vi "Read Bytes by Value.vi"(8 "Error In":errorcluster, 10 "Count":u64, 11 "Reader In":refnum<class "Reader.lvclass">) -> (0 "Error Out":errorcluster, 2 "Bytes":u8[](array[numeric]), 3 "Reader Out":refnum<class "Reader.lvclass">)   [LabVIEW 2018, in "Toolkit.lvlib" / "Reader.lvclass"]
uses:
  Reader.lvclass
  Reader.lvclass/Reader.ctl
  Public/Status/Read Status.vi
  Public/Status/Read Status Message.vi
  Public/Status/Read Is Error.vi
  Utility/Status Code.vi
  <vilib>/Utility/error.llb/Error Cluster From Error Code.vi
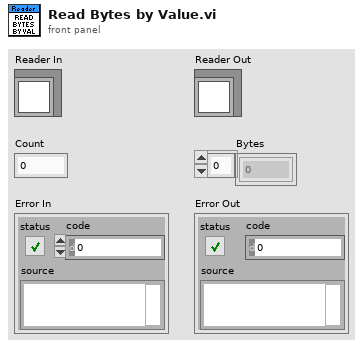
[diagram p1: front panel]
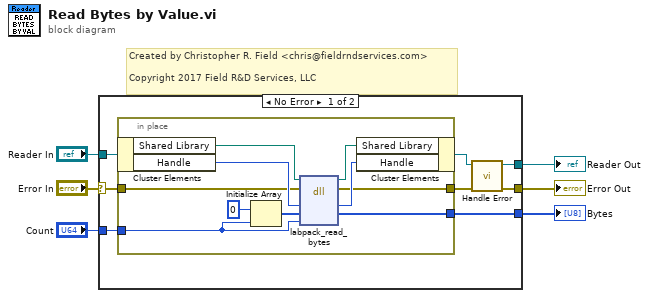
[diagram p0: block diagram]
diagram:
  # "Created by Christopher R. Field <chris@fieldrndservices.com>\n\nCopyright 2017 Field R&D Services, LLC"
  n1 = case shown="No Error" "Error In" {
    selector: "Error In" -> [w13 w25]
    tunnel: "Reader In" -> [w14 w26]
    tunnel: [w9 w25] -> w4
    tunnel: [w11 w26] -> w3
    tunnel: "Count" -> [w8 _]
    tunnel: [w7 _] -> w1
    frame No Error {
      n2 = in-place {
        in-place-border: w13 -> [w20]
        in-place-border: [w19] -> w10
        in-place-border: w8 -> [w17]
        in-place-border: [w15] -> w7
        n3 = in-place-cluster #1(w14) -> ("Shared Library"=w24:path, "Handle"=w22:u64)
        n4 = Initialize Array(u8 0, w17) -> (w16:u8[])
        n5 = dll-call lib="D:/Users/cfield/Code/MessagePack/LabPack/LabVIEW/trunk/src/LabPack/Private/labpack-x64.dll" fn="labpack_read_bytes"(path in=w24, error in=w20, "reader"=w22, "data"=w16, "count"=w17) -> (path out=w23:path, error out=w19:errorcluster, "reader"=w21:u64, "data"=w15:u8[])  [unwired: 3 in]
        n6 = in-place-cluster #1("Shared Library"=w23, "Handle"=w21) -> (w12:refnum<class "Reader.lvclass">)
      }
      n7 = call "Handle Error.vi"("Error In"=w10, "Reader In"=w12) -> ("Error Out"=w9:errorcluster, "Reader Out"=w11:refnum<class "Reader.lvclass">)  [unwired: 8 in]
    }
    frame Error {
    }
  }
  "Error Out" <- w4
  "Reader Out" <- w3
  "Bytes" <- w1
